vi "Logging Update - Boolean.vi"(4 "error in (no error)":errorcluster, 5 "Value":bool, 6 "Name":string, 7 "LoggingDevRef":T1) -> (0 "error out":errorcluster, 3 "LoggingDevRef":T1)   [LabVIEW 2012, in "femtoRoboLib.lvlib"]
doc: "Set <b>Name</b> to the boolean <b>Value</b> at specified Logging reference. This simply updates the cache, and does not automatically write the log file."
uses:
  femtoRoboLib.lvlib
  Controls/LoggingDevRef.ctl
  Controls/Log Entry - Converted.ctl
  Controls/Logging Cache - Mode.ctl
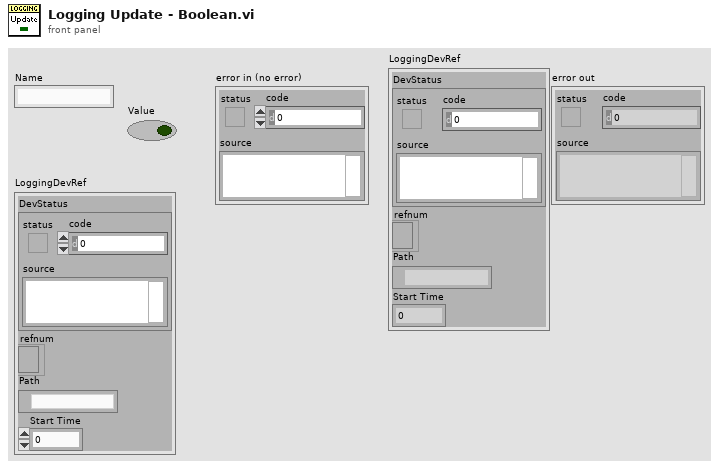
[diagram p1: front panel]
types:
  T1 = typedef "femtoRoboLib.lvlib/LoggingDevRef.ctl" = cluster{"DevStatus":errorcluster, "refnum":refnum<file>, "Path":path, "Start Time":u32}
  T2 = typedef "Logging Cache - Mode.ctl" = enum16{"Set", "Get All", "Get Unsaved", "Get Unsaved and Clear", "Get New", "Get New and Clear"}
  T3 = enum16{"Boolean", "Numeric", "String", "Boolean Array", "Numeric Array", "String Array"}
  T4 = typedef "femtoRoboLib.lvlib/Log Entry - Converted.ctl" = cluster{"Name":string, "Type":enum16{"Boolean", "Numeric", "String", "Boolean Array", "Numeric Array", "String Array"}, "Value":string, "ID":u32}
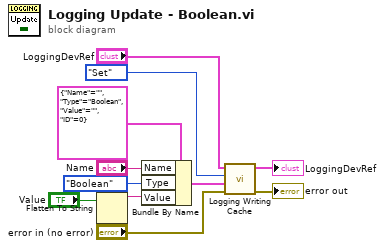
[diagram p0: block diagram]
diagram:
  n1 = Flatten To String(anything="Value") -> (data string=w10:string)  [unwired: 3 in, 2 out]
  n2 = Bundle By Name(cluster=T4 {"Name"="", "Type"=enum."Boolean", "Value"="", "ID"=0} ("Log Variable"), "Name"="Name", "Type"=T3."Boolean", "Value"=w10) -> (w7:T4)
  n3 = call "Logging Writing Cache.vi"("error in (no error)"="error in (no error)", "Variable"=w7, "Mode"=Logging_Cache_-_Mode."Set", "LoggingDevRef"="LoggingDevRef") -> ("error out"=→"error out":errorcluster, "LoggingDevRef"=→"LoggingDevRef":T1)  [unwired: 1 in, 1 out]
